vi "LWXPS_ColseAllOtherSockets.vi"(6 "LabVIEW error IN":errorcluster, 9 "XPS Reference IN":refnum<k24>) -> (0 "LabVIEW error OUT":errorcluster, 1 "XPS Error String":string, 2 "Returned error code":i32, 3 "XPS Reference OUT":refnum<k24>)   [LabVIEW 2013]
uses:
  D:/XPSQ8_LabView_Library/Development/Source/Dll/Newport.XPS.CommandInterface.dll
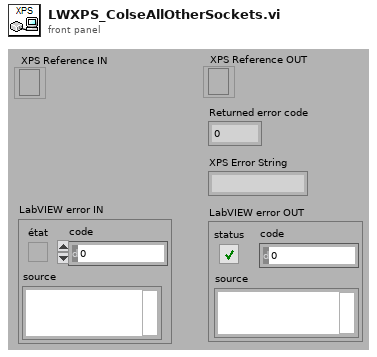
[diagram p1: front panel]
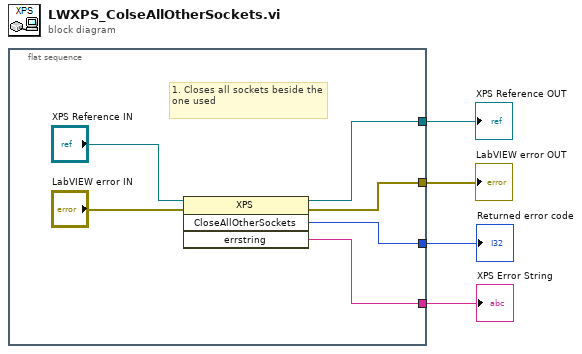
[diagram p0: block diagram]
diagram:
  n1 = flat-sequence {
    tunnel: [w7] -> w4
    tunnel: [w8] -> w3
    tunnel: [w6] -> w2
    tunnel: [w5] -> w1
    frame #0 {
      # "1. Closes all sockets beside the one used"
      n2 = invoke class="XPS" method="CloseAllOtherSockets"(reference="XPS Reference IN", error in="LabVIEW error IN") -> (reference out=w7:refnum<k24>, error out=w8:errorcluster, "CloseAllOtherSockets"=w5:i32, "errstring"=w6:string)  [unwired: 2 in]
    }
  }
  "XPS Reference OUT" <- w4
  "LabVIEW error OUT" <- w3
  "XPS Error String" <- w2
  "Returned error code" <- w1
